vi "CRYWindow WAIT CLOSE FRAME.vi"(10 "vi reference":refnum<vi>) -> ()   [LabVIEW 2013]
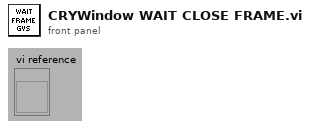
[diagram p1: front panel]
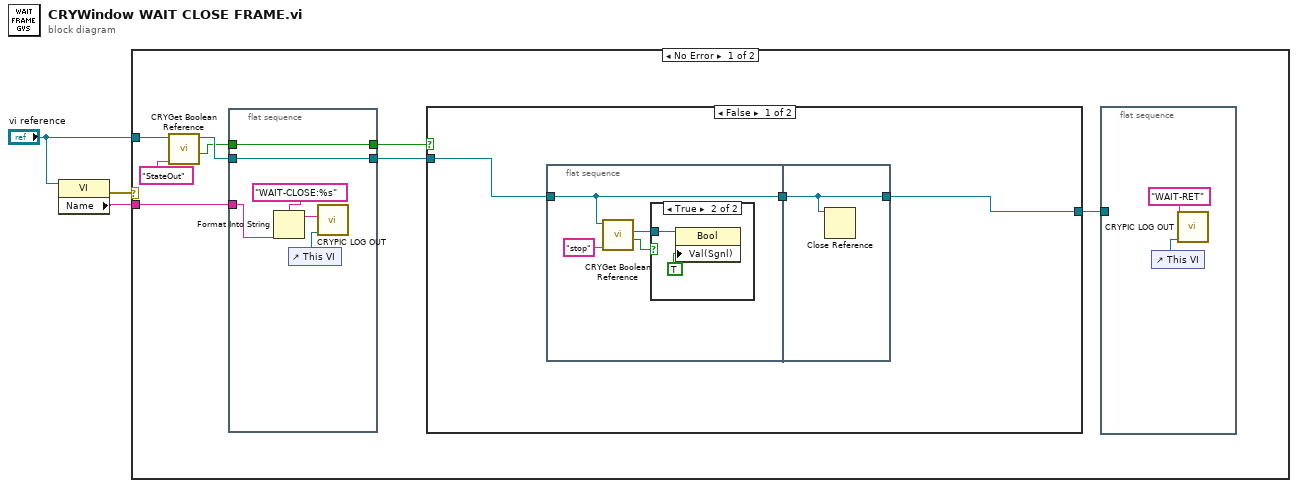
[diagram p0: block diagram]
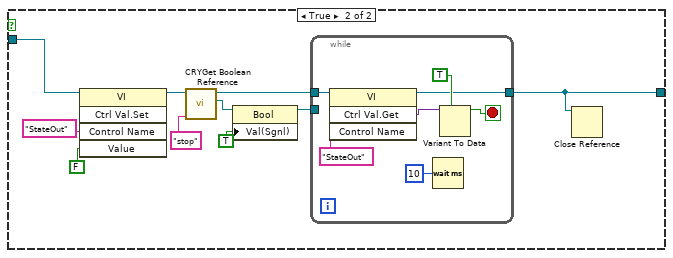
[diagram p3: hidden frame]
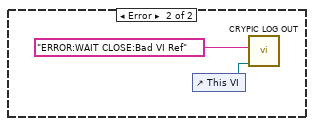
[diagram p4: hidden frame]
diagram:
  n1 = property class="VI"(reference="vi reference") -> (error out=w3:errorcluster, "Name"=w1:string)  [unwired: 1 in, 1 out]
  n2 = case shown="No Error" w3 {
    tunnel: "vi reference" -> [w5 _]
    tunnel: w1 -> [w4 _]
    frame No Error {
      n3 = call "CRYGet Boolean Reference.vi"("Label Name"="StateOut", "VI Refnum"=w5) -> ("Exist?"=w7:bool, "VI Refnum Out"=w8:refnum<vi>)  [unwired: 7 in, 1 out]
      n4 = flat-sequence {
        tunnel: [w44] -> w11
        tunnel: w8 -> [w44]
        tunnel: [w46] -> w6
        tunnel: w7 -> [w46]
        tunnel: w4 -> [w42]
        frame #0 {
          n5 = Format Into String(format string="WAIT-CLOSE:%s", w42) -> (resulting string=w43:string)  [unwired: 2 in, 1 out]
          n6 = control-ref of="This VI"() -> (w41:refnum<vi>)
          n7 = call "CRYPIC LOG OUT.vi"("pVIRef"=w41, "sData"=w43) -> ()  [unwired: 10 in]
        }
      }
      n8 = case shown="False" w6 {
        tunnel: w11 -> [w14 w24]
        tunnel: [w12 w22] -> w10
        frame False {
          n9 = flat-sequence {
            tunnel: w14 -> [w16]
            tunnel: [w16] -> w13
            tunnel: w13 -> [w21]
            tunnel: [w21] -> w12
            frame #0 {
              n10 = call "CRYGet Boolean Reference.vi"("Label Name"="stop", "VI Refnum"=w16) -> ("Exist?"=w15:bool, "Boolean Ref"=w18:refnum<vi>)  [unwired: 7 in, 1 out]
              n11 = case shown="True" w15 {
                tunnel: w18 -> [_ w20]
                frame False {
                }
                frame True {
                  n12 = property class="Bool"(reference=w20, "Val(Sgnl)"=TRUE) -> ()  [unwired: 1 in, 2 out]
                }
              }
            }
            frame #1 {
              n13 = Close Reference(reference=w21) -> ()  [unwired: 1 in, 1 out]
            }
          }
        }
        frame True {
          n14 = invoke class="VI" method="Ctrl Val.Set"(reference=w24, "Control Name"="StateOut", "Value"=FALSE) -> (reference out=w26:refnum<vi>)  [unwired: 2 in, 4 out]
          n15 = call "CRYGet Boolean Reference.vi"("Label Name"="stop", "VI Refnum"=w26) -> ("Boolean Ref"=w29:refnum<vi>, "VI Refnum Out"=w25:refnum<vi>)  [unwired: 7 in, 1 out]
          n16 = property class="Bool"(reference=w29, "Val(Sgnl)"=TRUE) -> (reference out=w23:refnum<vi>)  [unwired: 1 in, 1 out]
          n17 = while {
            tunnel: w25 -> [w37]
            tunnel: [w33] -> w22
            tunnel: w23 -> [_]
            stop <- w34 stop-if-true
            n18 = invoke class="VI" method="Ctrl Val.Get"(reference=w37, "Control Name"="StateOut") -> (reference out=w33:refnum<vi>, "Get Control Value Variant"=w36:variant)  [unwired: 2 in, 2 out]
            n19 = Wait (ms)(milliseconds to wait=u32 10) -> ()  [unwired: 1 out]
            n20 = Variant To Data(type=TRUE, Variant=w36) -> (data=w34:bool)  [unwired: 1 in, 1 out]
          }
          n21 = Close Reference(reference=w22) -> ()  [unwired: 1 in, 1 out]
        }
      }
      n22 = flat-sequence {
        tunnel: w10 -> [_]
        frame #0 {
          n23 = control-ref of="This VI"() -> (w39:refnum<vi>)
          n24 = call "CRYPIC LOG OUT.vi"("pVIRef"=w39, "sData"="WAIT-RET") -> ()  [unwired: 10 in]
        }
      }
    }
    frame Error {
      n25 = control-ref of="This VI"() -> (w47:refnum<vi>)
      n26 = call "CRYPIC LOG OUT.vi"("pVIRef"=w47, "sData"="ERROR:WAIT CLOSE:Bad VI Ref" ("format string")) -> ()  [unwired: 10 in]
    }
  }
